vi "3.2.1.vi"() -> ()   [LabVIEW 2023]
panel:
  out "Analog Input AI0 (V)":dbl
  in  "Analog Output AO0 (V)":dbl
  # "THING GOES HERE"
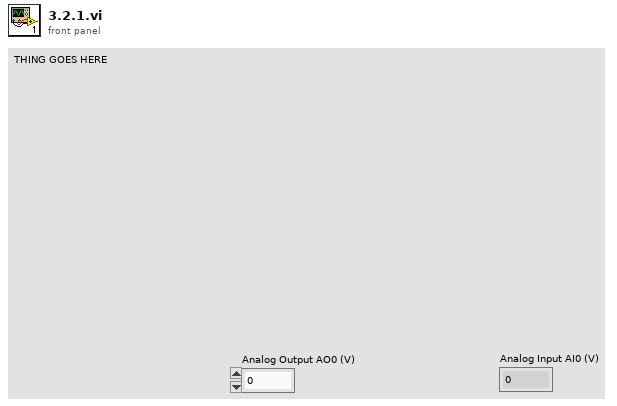
[diagram p1: front panel]
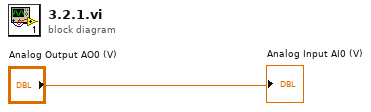
[diagram p0: block diagram]
diagram:
  "Analog Input AI0 (V)" <- "Analog Output AO0 (V)"
